vi "UpdateAttackMap.vi"(4 "Attacked?":bool, 7 "Position":cluster{"Column":i32, "Row":i32}, 11 "AttackMap DVR In":T1) -> (3 "AttackMap DVR Out":T1)   [LabVIEW 2017, in "Atom.lvclass"]
uses:
  Atom.lvclass
  AttackMap DVR.ctl
  Common/Position.ctl
  Common/Common.lvlib
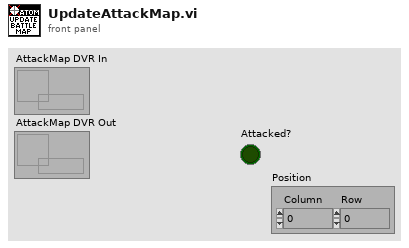
[diagram p1: front panel]
types:
  T1 = typedef "Atom.lvclass/AttackMap DVR.ctl" = refnum<data-value>
  T2 = typedef "Common.lvlib/Position.ctl" = cluster{"Column":i32, "Row":i32}
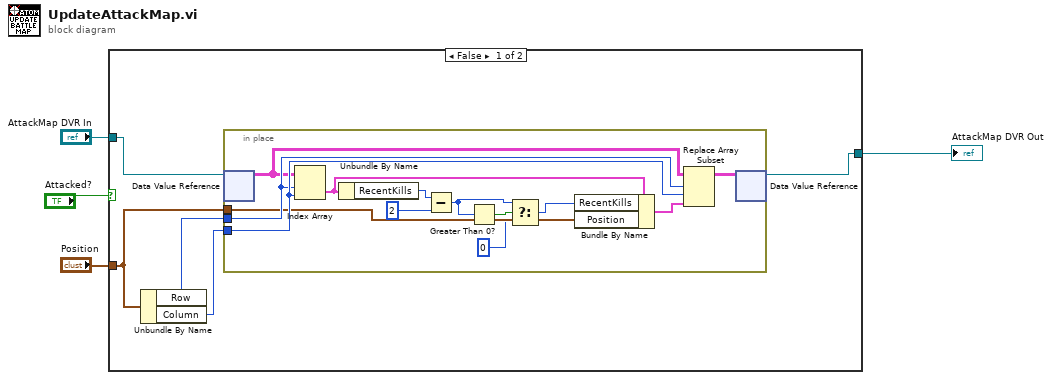
[diagram p0: block diagram]
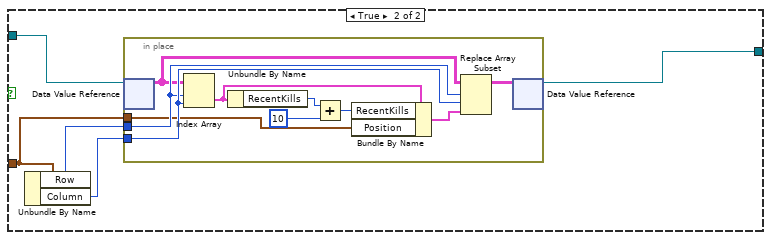
[diagram p2: hidden frame]
diagram:
  n1 = case shown="False" "Attacked?" {
    tunnel: "AttackMap DVR In" -> [w9 w27]
    tunnel: "Position" -> [w5 w23]
    tunnel: [w8 w24] -> w2
    frame False {
      n2 = Unbundle By Name(w5) -> ("Row"=w6:i32, "Column"=w7:i32)
      n3 = in-place {
        in-place-border: w6 -> [w19]
        in-place-border: w7 -> [w20]
        in-place-border: w5 -> [w16]
        n4 = in-place-dvr #1(w9) -> (w18:cluster{"RecentKills":i32, "Position":T2}[][])  [unwired: 1 out]
        n5 = Index Array(array=w18, index (row)=w19, index (col)=w20) -> (element=w22:cluster{"RecentKills":i32, "Position":T2})
        n6 = Unbundle By Name(w22) -> ("RecentKills"=w15:i32)
        n7 = Subtract(x=w15, y=2 ("x")) -> (x-y=w11:i32)
        n8 = Greater Than 0?(x=w11) -> (x > 0?=w13:bool)
        n9 = Select(t=w11, s=w13, f=0 ("x")) -> (s? t:f=w10:i32)
        n10 = Bundle By Name(cluster=w22, "RecentKills"=w10, "Position"=w16) -> (w21:cluster{"RecentKills":i32, "Position":T2})
        n11 = Replace Array Subset(array=w18, new element=w21, index (row)=w19, index (col)=w20) -> (w17:cluster{"RecentKills":i32, "Position":T2}[][])
        n12 = in-place-dvr #1(w17) -> (w8:T1)  [unwired: 1 out]
      }
    }
    frame True {
      n13 = Unbundle By Name(w23) -> ("Row"=w26:i32, "Column"=w25:i32)
      n14 = in-place {
        in-place-border: w26 -> [w33]
        in-place-border: w25 -> [w34]
        in-place-border: w23 -> [w30]
        n15 = in-place-dvr #2(w27) -> (w32:cluster{"RecentKills":i32, "Position":T2}[][])  [unwired: 1 out]
        n16 = Index Array(array=w32, index (row)=w33, index (col)=w34) -> (element=w37:cluster{"RecentKills":i32, "Position":T2})
        n17 = Unbundle By Name(w37) -> ("RecentKills"=w29:i32)
        n18 = Add(x=w29, y=10 ("x")) -> (x+y=w36:i32)
        n19 = Bundle By Name(cluster=w37, "RecentKills"=w36, "Position"=w30) -> (w35:cluster{"RecentKills":i32, "Position":T2})
        n20 = Replace Array Subset(array=w32, new element=w35, index (row)=w33, index (col)=w34) -> (w31:cluster{"RecentKills":i32, "Position":T2}[][])
        n21 = in-place-dvr #2(w31) -> (w24:T1)  [unwired: 1 out]
      }
    }
  }
  "AttackMap DVR Out" <- w2
